vi "writeGainXML.vi"(8 "error in (no error)":errorcluster, 10 "NativeXML in":refnum<class "NativeXML.lvclass">, 11 "PixelflySettings in":refnum<class "PixelflySettings.lvclass">) -> (0 "error out":errorcluster, 2 "NativeXML out":refnum<class "NativeXML.lvclass">, 3 "PixelflySettings out":refnum<class "PixelflySettings.lvclass">)   [LabVIEW 2011, in "Tools.lvlib" / "Settings.lvlib" / "PixelflySettings.lvclass"]
uses:
  PixelflySettings.lvclass
  NativeXML/NativeXML.lvclass
  PixelflySettings.lvclass/PixelflySettings.ctl
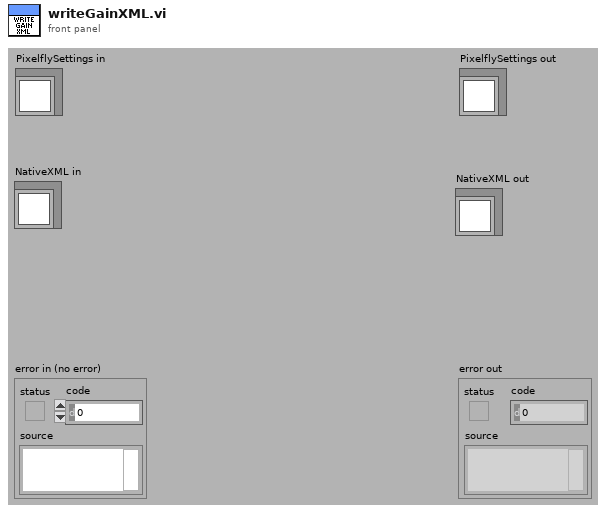
[diagram p1: front panel]
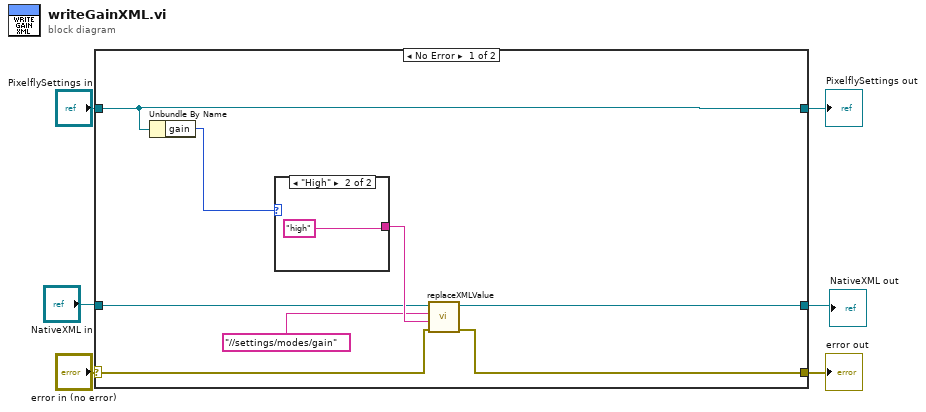
[diagram p0: block diagram]
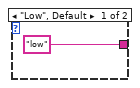
[diagram p2: hidden frame]
diagram:
  n1 = case shown="No Error" "error in (no error)" {
    selector: "error in (no error)" -> [w10 w18]
    tunnel: [w9 w18] -> w5
    tunnel: [w11 w17] -> w3
    tunnel: "PixelflySettings in" -> [w11 w17]
    tunnel: "NativeXML in" -> [w8 _]
    tunnel: [w7 _] -> w1
    frame No Error {
      n2 = Unbundle By Name(w11) -> ("gain"=w14:enum16{"Low", "High"})
      n3 = case shown="\"High\"" w14 {
        tunnel: ["low" "high"] -> w13
        frame "Low", Default {
        }
        frame "High" {
        }
      }
      n4 = call "replaceXMLValue.vi"("error in (no error)"=w10, "value"=w13, "replace in"="//settings/modes/gain", "NativeXML in"=w8) -> ("error out"=w9:errorcluster, "NativeXML out"=w7:refnum<class "NativeXML.lvclass">)  [unwired: 6 in]
    }
    frame Error {
    }
  }
  "error out" <- w5
  "PixelflySettings out" <- w3
  "NativeXML out" <- w1
